vi "WritePoint.vi"(2 "FullPath":path, 3 "TimeToWrite":u32) -> (0 "SampleChunk":dbl[](array[numeric]), 1 "Frequency":dbl)   [LabVIEW 2010]
uses:
  Instance           8 18Saved   WritePoint .vi
  Instance           7 18Saved   WritePoint .vi
  Instance           5 18Saved   WritePoint .vi
  Instance           9 18Saved   WritePoint .vi
  Instance           6 18Saved   WritePoint .vi
  Instance           4 18Saved   WritePoint .vi
  Instance           3 18Saved   WritePoint .vi
  Instance           2 18Saved   WritePoint .vi
panel:
  out "Scaled Signals":dynamicdata(graph)
  out "error out 3":errorcluster
  out "error out 2":errorcluster
  out "error out":errorcluster
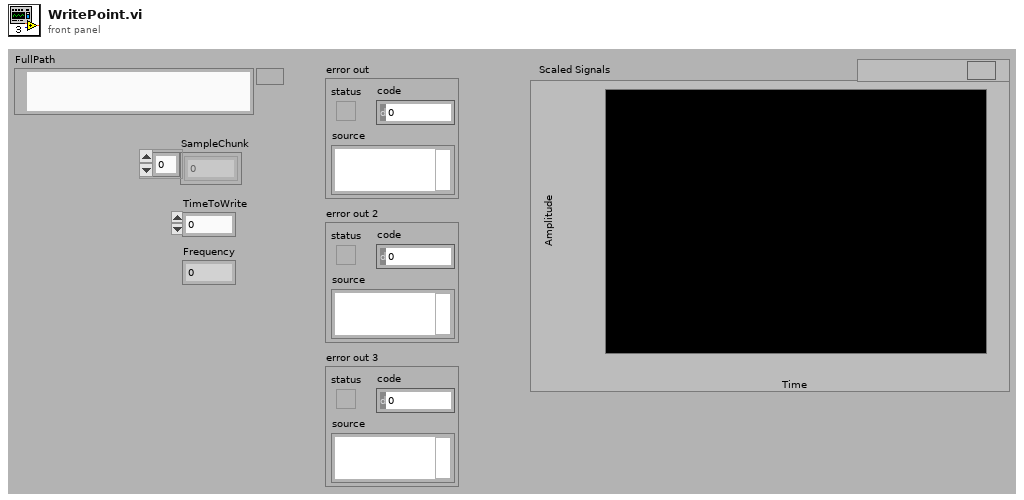
[diagram p1: front panel]
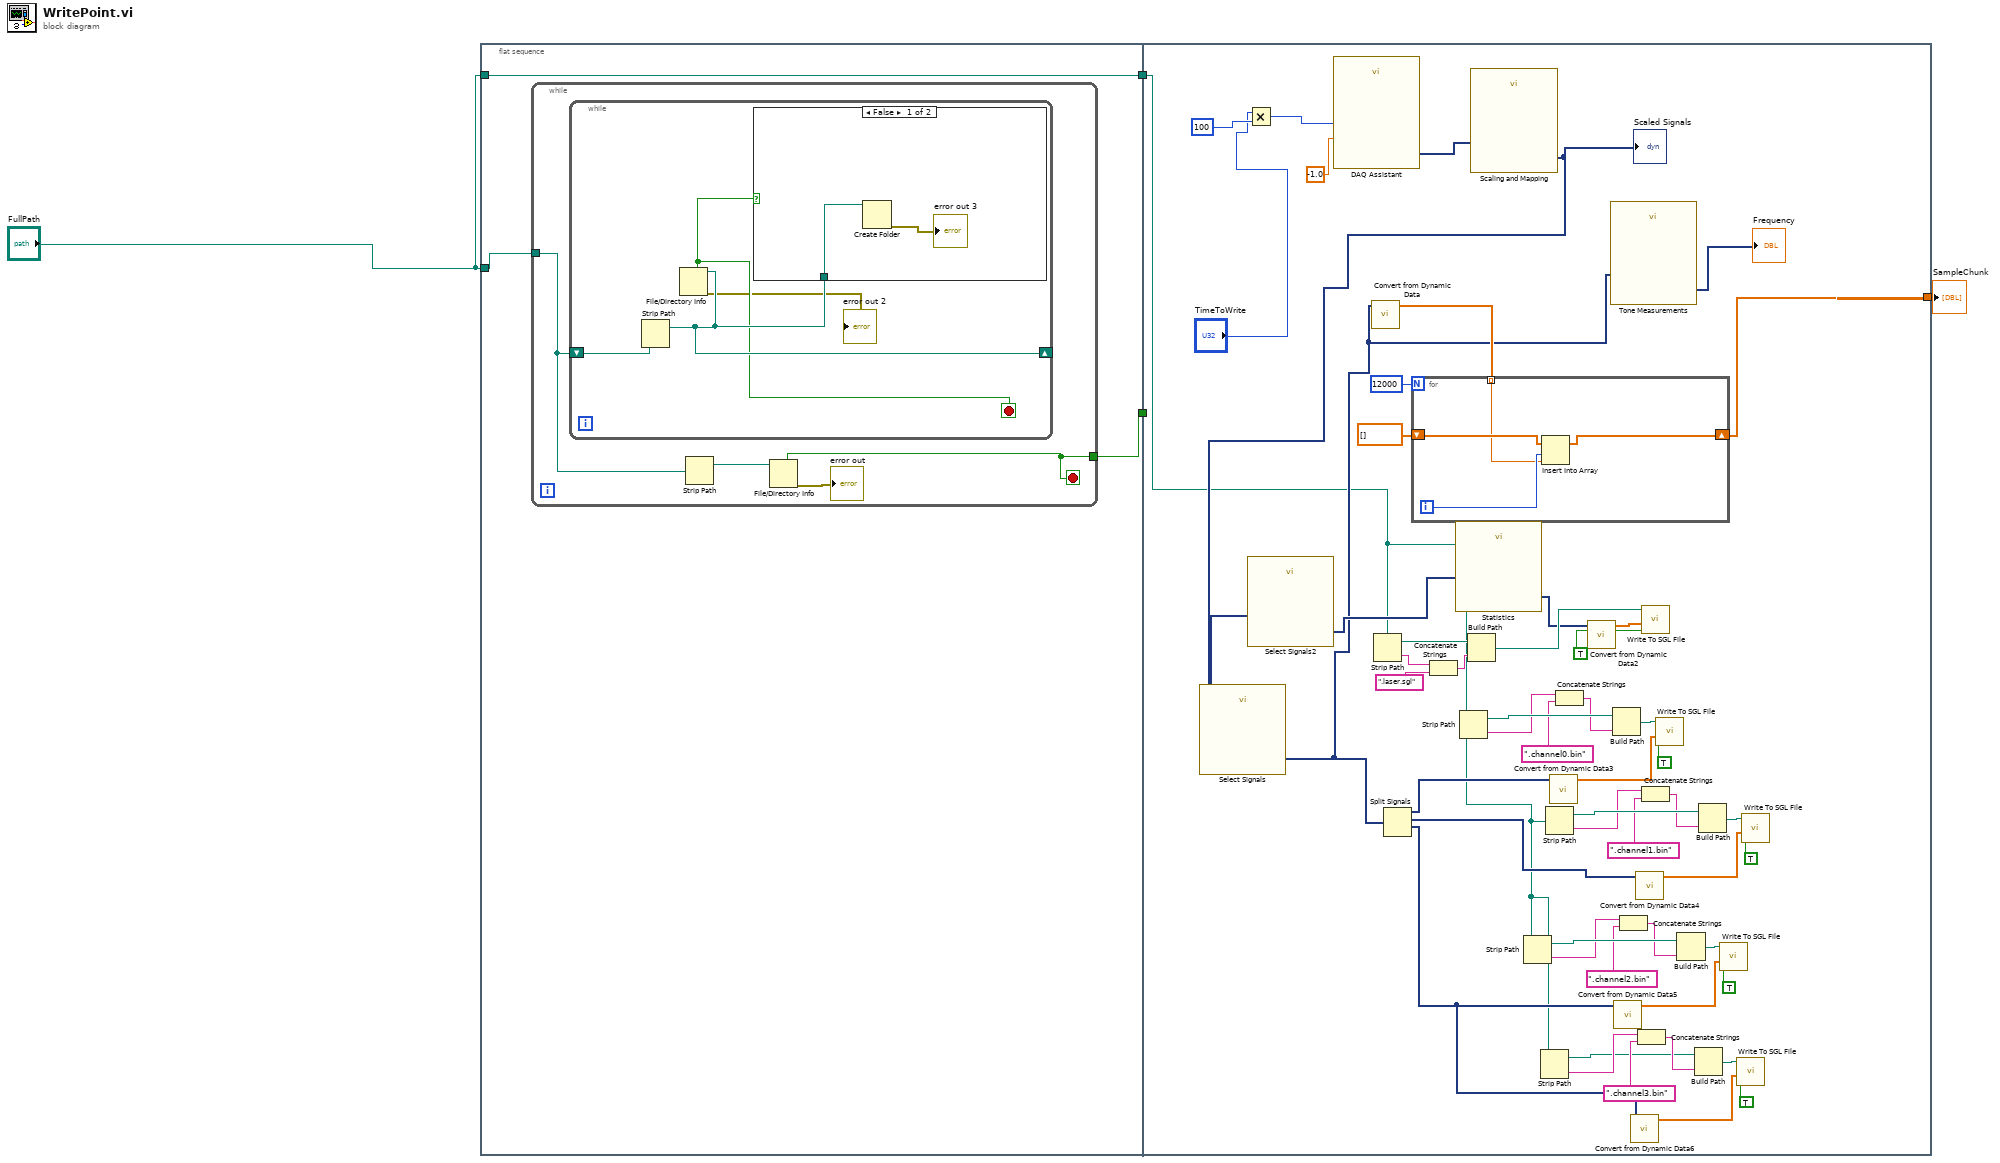
[diagram p0: block diagram]
diagram:
  n1 = flat-sequence {
    tunnel: "FullPath" -> [w7]
    tunnel: [w6] -> w4
    tunnel: "FullPath" -> [w6]
    tunnel: [w5] -> w2
    tunnel: w4 -> [w18]
    tunnel: w2 -> [_]
    tunnel: [w67] -> w1
    frame #0 {
      n2 = while {
        tunnel: w7 -> [w10]
        tunnel: [w9] -> w5
        stop <- w9 stop-if-true
        n3 = while {
          shift-right: [w14] -> _
          shift-left: w10 -> [w15]
          stop <- w13 stop-if-true
          n4 = Strip Path(path=w15) -> (stripped path=w14:path)  [unwired: 1 out]
          n5 = File/Directory Info(path=w14) -> (directory=w13:bool, error out=→"error out 2":errorcluster)  [unwired: 1 in, 5 out]
          n6 = case shown="False" w13 {
            tunnel: w14 -> [w17 _]
            frame False {
              n7 = Create Folder(path (use dialog)=w17) -> (error out=→"error out 3":errorcluster)  [unwired: 2 in, 2 out]
            }
            frame True {
            }
          }
        }
        n8 = Strip Path(path=w10) -> (stripped path=w11:path)  [unwired: 1 out]
        n9 = File/Directory Info(path=w11) -> (directory=w9:bool, error out=→"error out":errorcluster)  [unwired: 1 in, 5 out]
      }
    }
    frame #1 {
      n10 = Multiply(x="TimeToWrite", y=u32 100) -> (x*y=w63:u32)
      n11 = call "DAQ Assistant"("number of samples"=w63, "timeout (s)"=-1.0 ("timeout (sec)")) -> ("data"=w65:dynamicdata)  [unwired: 15 in, 2 out]
      n12 = Strip Path(path=w18) -> (stripped path=w60:path, name=w59:string)
      n13 = Concatenate Strings(w59, ".laser.sgl" ("string")) -> (w57:string)
      n14 = Strip Path(path=w18) -> (stripped path=w46:path, name=w45:string)
      n15 = Build Path(base path=w60, name or relative path=w57) -> (appended path=w56:path)
      n16 = call "Scaling and Mapping"("Signals"=w65) -> ("Scaled Signals"=w54:dynamicdata)  [unwired: 9 in, 1 out]
      "Scaled Signals" <- w54
      n17 = call "Select Signals"("Signals"=w54) -> ("Signal Out"=w50:dynamicdata)  [unwired: 9 in, 1 out]
      n18 = call "Select Signals2"("Signals"=w54) -> ("Signal Out"=w53:dynamicdata)  [unwired: 9 in, 1 out]
      n19 = call "Convert from Dynamic Data"("Dynamic Data Type"=w50) -> ("Array"=w69:dbl[])  [unwired: 3 in]
      n20 = Split Signals(w50) -> (w47:dynamicdata, w34:dynamicdata, w19:dynamicdata)  [unwired: 4 in, 1 out]
      n21 = for {
        N: 12000 -> [_]
        tunnel: w69 -> [w71] mode=indexing
        shift-right: [w72] -> w67
        shift-left: dbl[] [] -> [w73]
        i -> [w74]
        n22 = Insert Into Array(array=w73, index=w74, new element=w71) -> (w72:dbl[])
      }
      n23 = call "Statistics"("Signals"=w53) -> ("Arithmetic Mean"=w52:dynamicdata)  [unwired: 25 in, 1 out]
      n24 = Strip Path(path=w18) -> (stripped path=w31:path, name=w30:string)
      n25 = Strip Path(path=w18) -> (stripped path=w22:path, name=w23:string)
      n26 = Strip Path(path=w18) -> (stripped path=w39:path, name=w38:string)
      n27 = call "Convert from Dynamic Data3"("Dynamic Data Type"=w47) -> ("Array"=w48:dbl[])  [unwired: 3 in]
      n28 = Concatenate Strings(w45, ".channel0.bin" ("string")) -> (w43:string)
      n29 = call "Convert from Dynamic Data2"("Dynamic Data Type"=w52) -> ("Array"=w51:dbl[])  [unwired: 3 in]
      n30 = call "Tone Measurements"("Signals"=w50) -> ("Frequency"=→"Frequency":dynamicdata)  [unwired: 9 in, 1 out]
      n31 = Build Path(base path=w46, name or relative path=w43) -> (appended path=w42:path)
      n32 = call "Convert from Dynamic Data5"("Dynamic Data Type"=w19) -> ("Array"=w32:dbl[])  [unwired: 3 in]
      n33 = Concatenate Strings(w30, ".channel2.bin" ("string")) -> (w28:string)
      n34 = call "Convert from Dynamic Data6"("Dynamic Data Type"=w19) -> ("Array"=w21:dbl[])  [unwired: 3 in]
      n35 = call "Convert from Dynamic Data4"("Dynamic Data Type"=w34) -> ("Array"=w40:dbl[])  [unwired: 3 in]
      n36 = Concatenate Strings(w23, ".channel3.bin" ("string")) -> (w25:string)
      n37 = call <vilib>:"Write To SGL File.vi"("append to file? (new file:F)"=TRUE, "1D array"=w51, "file path (dialog if empty)"=w56) -> ()  [unwired: 4 in, 1 out]
      n38 = Concatenate Strings(w38, ".channel1.bin" ("string")) -> (w36:string)
      n39 = call <vilib>:"Write To SGL File.vi"("append to file? (new file:F)"=TRUE, "1D array"=w48, "file path (dialog if empty)"=w42) -> ()  [unwired: 4 in, 1 out]
      n40 = Build Path(base path=w31, name or relative path=w28) -> (appended path=w27:path)
      n41 = Build Path(base path=w22, name or relative path=w25) -> (appended path=w26:path)
      n42 = Build Path(base path=w39, name or relative path=w36) -> (appended path=w35:path)
      n43 = call <vilib>:"Write To SGL File.vi"("append to file? (new file:F)"=TRUE, "1D array"=w32, "file path (dialog if empty)"=w27) -> ()  [unwired: 4 in, 1 out]
      n44 = call <vilib>:"Write To SGL File.vi"("append to file? (new file:F)"=TRUE, "1D array"=w21, "file path (dialog if empty)"=w26) -> ()  [unwired: 4 in, 1 out]
      n45 = call <vilib>:"Write To SGL File.vi"("append to file? (new file:F)"=TRUE, "1D array"=w40, "file path (dialog if empty)"=w35) -> ()  [unwired: 4 in, 1 out]
    }
  }
  "SampleChunk" <- w1
